vi "State Exit Core.vi"(8 "error in (no error)":errorcluster, 11 "Context in":refnum<class "Context.lvclass">) -> (0 "error out":errorcluster, 3 "Context out":refnum<class "Context.lvclass">)   [LabVIEW 2021, in "Context.lvclass"]
uses:
  Context.lvclass
  Context.lvclass/Context.ctl
  State Pattern/State Pattern.lvclass
  C:/PPLs/Design-Patterns/State Pattern/Context/Context.lvclass
  C:/PPLs/Design-Patterns/State Pattern/State Pattern/State Pattern.lvclass
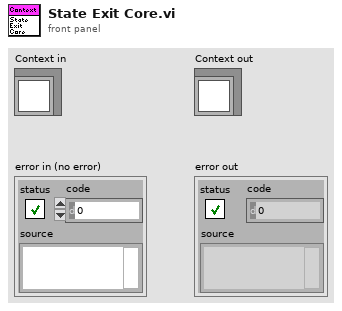
[diagram p1: front panel]
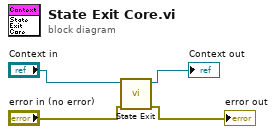
[diagram p0: block diagram]
diagram:
  n1 = call "State Exit.vi"("error in"="error in (no error)", "State Pattern in"="Context in") -> ("error out"=→"error out":errorcluster, "State Pattern out"=→"Context out":refnum<class "Context.lvclass">)  [unwired: 8 in]
